vi "libtrigger_all.vi"(8 "error in (no error)":errorcluster, 9 "Parameter":string, 10 "Function":string, 11 "input":i32) -> (0 "error out":errorcluster)   [LabVIEW 2015]
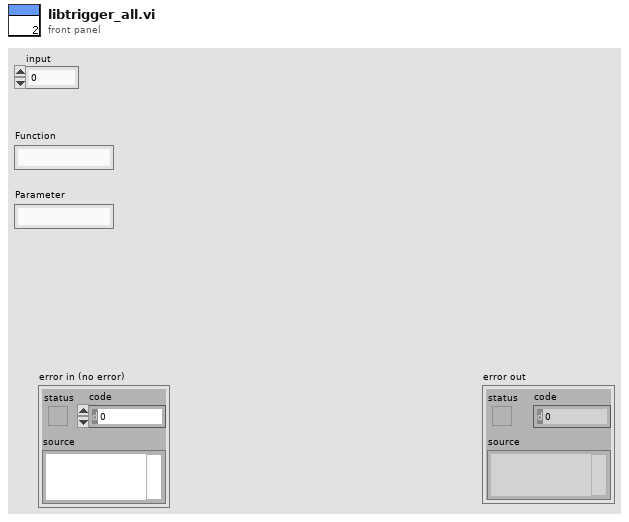
[diagram p1: front panel]
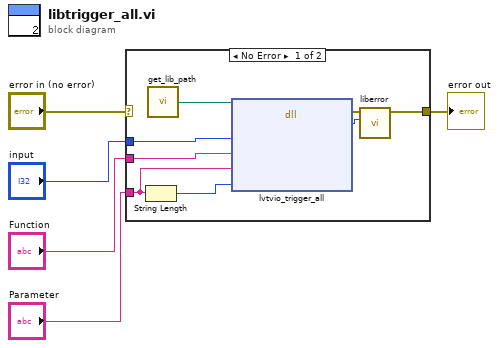
[diagram p0: block diagram]
diagram:
  n1 = case shown="No Error" "error in (no error)" {
    selector: "error in (no error)" -> [_ w14]
    tunnel: [w6 w14] -> w4
    tunnel: "Function" -> [w12 _]
    tunnel: "Parameter" -> [w11 _]
    tunnel: "input" -> [w9 _]
    frame No Error {
      n2 = String Length(string=w11) -> (length=w10:i32)
      n3 = call "get_lib_path.vi"() -> ("Path"=w13:path)
      n4 = dll-call lib="S:/thingiverselv/lib/liblvtvio.dll" fn="lvtvio_trigger_all"(path in=w13, "input"=w9, "function"=w12, "params"=w11, "params_size"=w10) -> (error out=w8:errorcluster, "return type"=w7:i32)  [unwired: 6 in, 1 out]
      n5 = call "liberror.vi"("tvio errors"=w7, "error in (no error)"=w8) -> ("error out"=w6:errorcluster)  [unwired: 9 in]
    }
    frame Error {
    }
  }
  "error out" <- w4
